vi "Cleanup.vi"(8 "error in (no error)":errorcluster, 11 "PanelManager in":refnum<class "PanelManager.lvclass">) -> (0 "error out":errorcluster)   [LabVIEW 2018, in "OOPanel.lvlib" / "PanelManager.lvclass"]
uses:
  PanelManager.lvclass
  PanelManager.lvclass/PanelManager.ctl
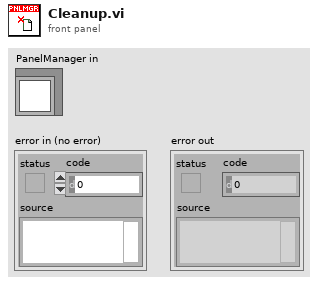
[diagram p1: front panel]
types:
  T1 = typedef "OOPanel.lvlib/PanelManager.lvclass/Ref Data.ctl" = cluster{"Panels":T2, "Subpanel Map":T3}
  T2 = typedef "OOPanel.lvlib/PanelManager.lvclass/Panels.ctl" = cluster{"Names":string[], "Instances":refnum<class "Panel.lvclass">[]}
  T3 = typedef "OOPanel.lvlib/PanelManager.lvclass/SubPanel Map.ctl" = cluster{"SubPanels":refnum<vi>[], "Panels":refnum<class "Panel.lvclass">[]}
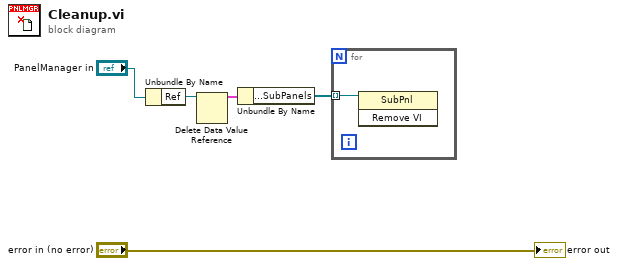
[diagram p0: block diagram]
diagram:
  n1 = Unbundle By Name("PanelManager in") -> ("Ref"=w3:refnum<data-value>)
  n2 = Delete Data Value Reference(data value reference=w3) -> (data value=w2:T1)  [unwired: 1 in, 1 out]
  n3 = Unbundle By Name(w2) -> ("Subpanel Map.SubPanels"=w1:refnum<vi>[])
  n4 = for {
    tunnel: w1 -> [w6] mode=indexing
    n5 = invoke class="SubPnl" method="Remove VI"(reference=w6) -> ()  [unwired: 2 in, 3 out]
  }
  "error out" <- "error in (no error)"
